vi "C884Config.vi"(0 "All axes? Refnum":refnum<vi>, 1 "Stage selection":T2={"Force?"=FALSE, "Dialog?"=TRUE, "Stages"=[]}, 2 "Position Refnum":refnum<vi>, 3 "Identification Refnum":refnum<vi>, 4 "Referencing successful Refnum":refnum<vi>, 5 "Host Addresss Refnum":refnum<vi>, 6 "Message Out Refnum":refnum<vi>, 7 "+/- mvt range Refnum":refnum<vi>, 8 "Axes to Move Refnum":refnum<vi>, 9 "Connected Axes Refnum":refnum<vi>, 10 "Referencing":T1={"Check FRF?"=TRUE, "Referencing mode"=[enum."FRF (-> FNL)", enum."FRF (-> FNL)", enum."FRF (-> FNL)", enum."FRF (-> FNL)", enum."FRF (-> FNL)", enum."FRF (-> FNL)"]}, 11 "Error OUT Refnum":refnum<vi>, 12 "En cours LED Refnum":refnum<vi>, 13 "LED Initialis. OK? Refnum":refnum<vi>) -> ()   [LabVIEW 2013]
panel:
  out "+/- movement\nrange":dbl[](array[numeric]) format="%.6f"
  out "error out":errorcluster
  out "Identification":string
  out "Referencing\nsuccessful?":bool[](array[boolean])
  out "Conn. \nAxes":string[](array[string])
  out "Position":dbl[](array[numeric]) format="%.6f"
  out "TCP/IP settings.Host address/name":string
  # "If yes:"
  # "If not:"
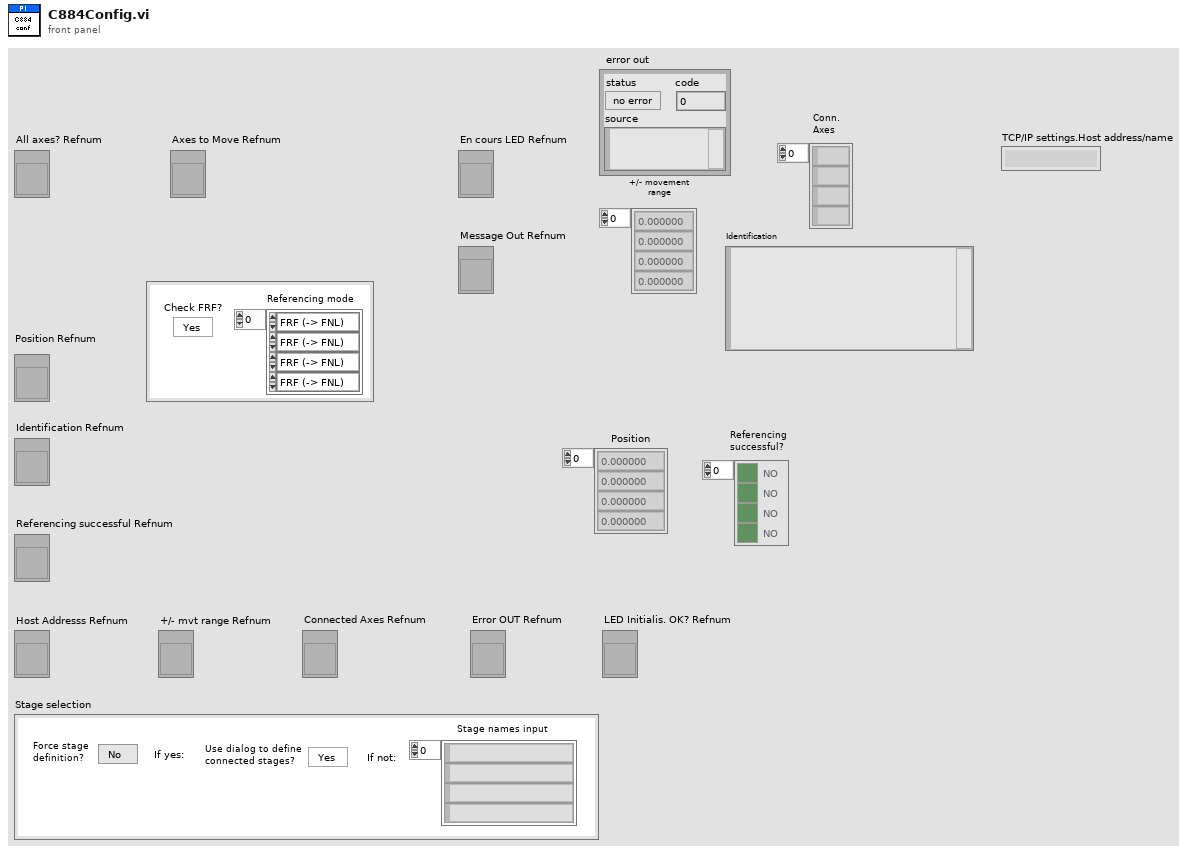
[diagram p1: front panel]
types:
  T1 = cluster{"Check FRF?":bool, "Referencing mode":enum16{"FRF (-> FNL)", "FRF", "FNL", "FPL", "RON OFF"}[]}
  T2 = cluster{"Force?":bool, "Dialog?":bool, "Stages":string[]}
  T3 = cluster{"RS232 settings":cluster{"Portnumber":i32, "Baudrate":u16}, "TCP/IP settings":cluster{"Host address/name":string, "Port":i32, "Board":i32, "TCP/IP Search?":bool}, "USB settings":cluster{"S/N":string, "USB Search?":bool}}
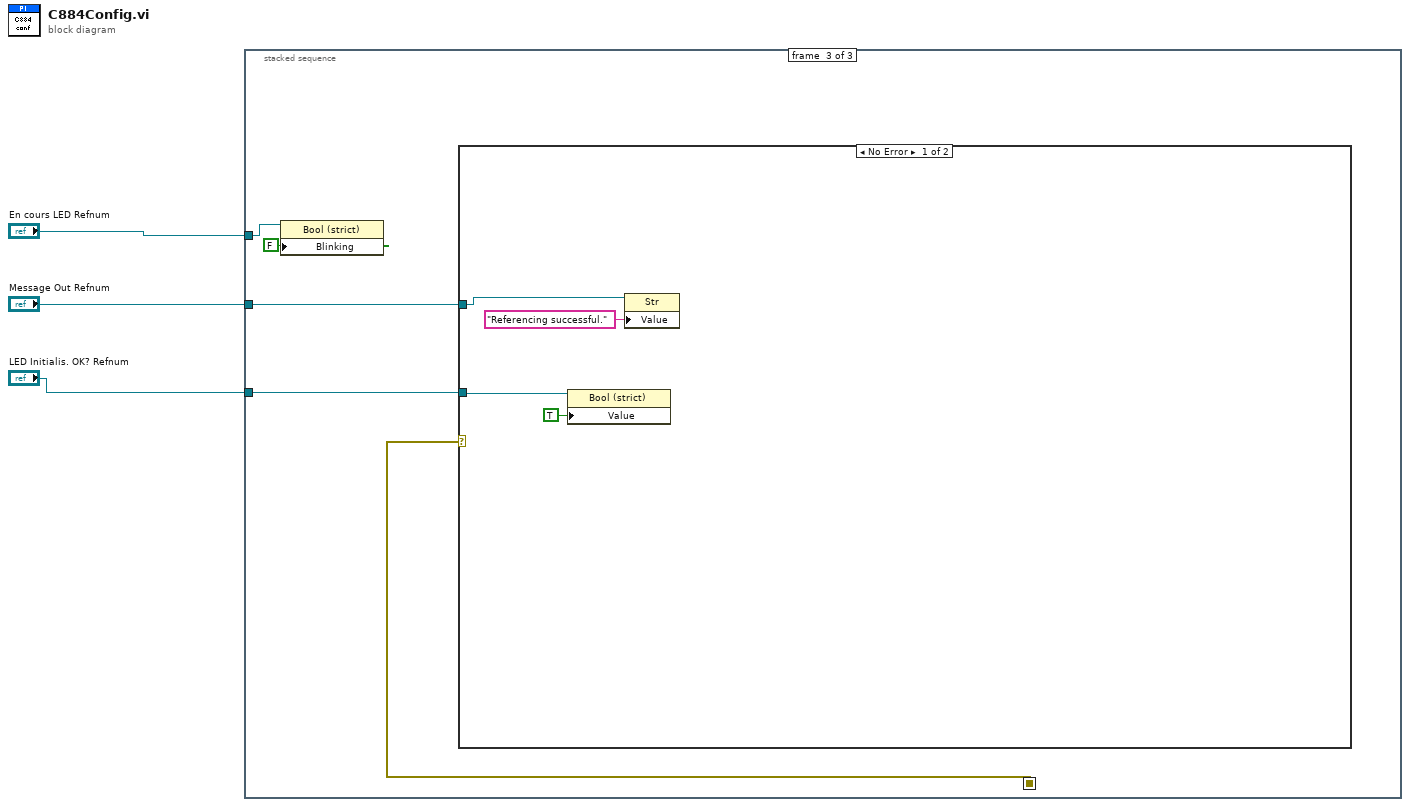
[diagram p0: block diagram]
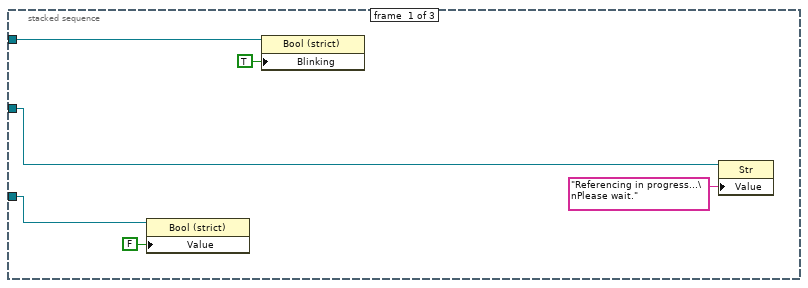
[diagram p2: hidden frame]
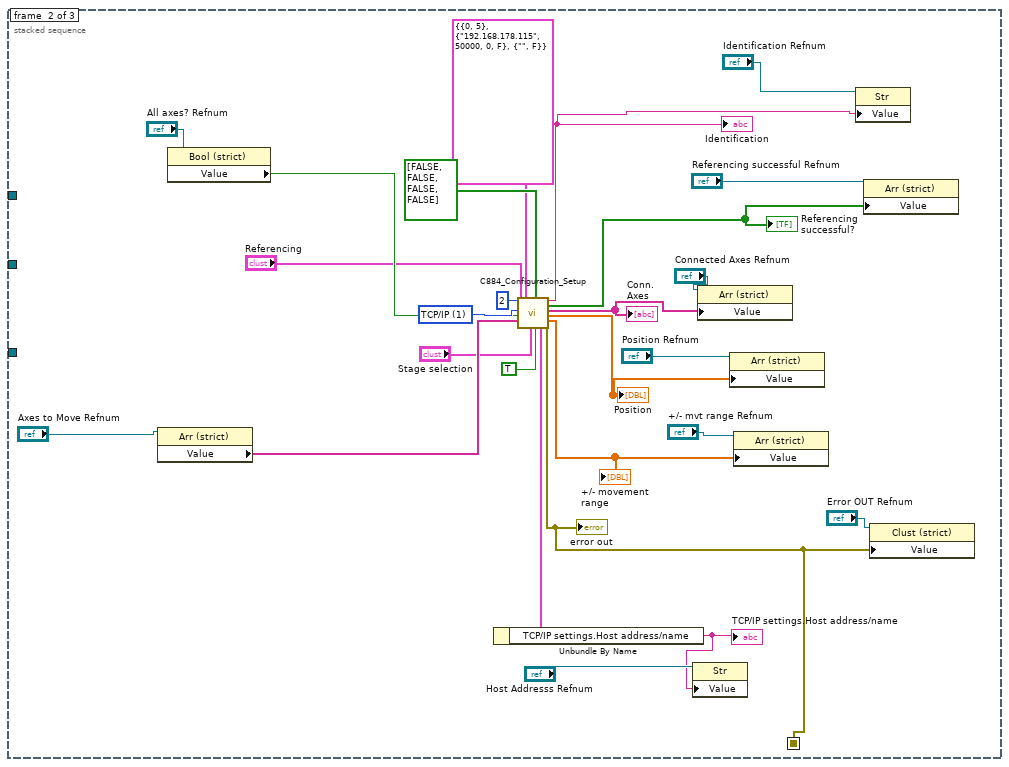
[diagram p3: hidden frame]
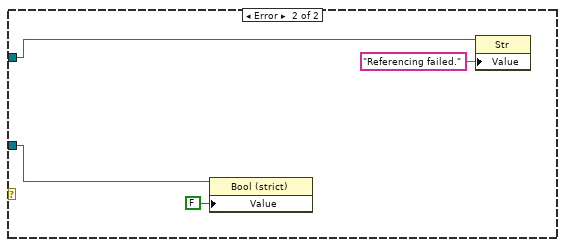
[diagram p4: hidden frame]
diagram:
  n1 = stacked-sequence {
    seq-local: [_ w14 _] -> [_ _ w38]
    tunnel: "En cours LED Refnum" -> [w8 _ w39]
    tunnel: "Message Out Refnum" -> [w7 _ w37]
    tunnel: "LED Initialis. OK? Refnum" -> [w5 _ w36]
    frame #0 {
      n2 = property class="Bool (strict)"(reference=w5, "Value"=FALSE) -> ()  [unwired: 1 in, 2 out]
      n3 = property class="Bool (strict)"(reference=w8, "Blinking"=TRUE) -> ()  [unwired: 1 in, 2 out]
      n4 = property class="Str"(reference=w7, "Value"="Referencing in progress...\nPlease wait.") -> ()  [unwired: 1 in, 2 out]
    }
    frame #1 {
      w32 = u16 1 items=["RS232", "TCP/IP", "USB"] ("Interface")
      n5 = property class="Arr (strict)"(reference="Axes to Move Refnum") -> ("Value"=w28:string[])  [unwired: 1 in, 2 out]
      n6 = property class="Bool (strict)"(reference="All axes? Refnum") -> ("Value"=w29:bool)  [unwired: 1 in, 2 out]
      n7 = call "C884_Configuration_Setup.vi"("System no."=2, "Referencing"="Referencing", "Interface"=w32, "All axes?"=w29, "Axes to move"=w28, "Interface settings"=T3 {"RS232 settings"={"Portnumber"=0, "Baudrate"=5}, "TCP/IP settings"={"Host address/name"="192.168.178.115", "Port"=50000, "Board"=0, "TCP/IP Search?"=FALSE}, "USB settings"={"S/N"="", "USB Search?"=FALSE}}, "Stage selection"="Stage selection", "Move to middle?"=bool[] [FALSE, FALSE, FALSE, FALSE], "Switch servo on?"=TRUE) -> ("Interface settings out"=w33:T3, "Identification"=w15:string, "Referencing\nsuccessful?"=w17:bool[], "Conn. \nAxes"=w19:string[], "Position"=w21:dbl[], "+/- movement\nrange"=w23:dbl[], "error out"=w14:errorcluster)  [unwired: 4 in]
      "Position" <- w21
      "Conn. \nAxes" <- w19
      "Referencing\nsuccessful?" <- w17
      "Identification" <- w15
      "error out" <- w14
      "+/- movement\nrange" <- w23
      n8 = Unbundle By Name(w33) -> ("TCP/IP settings.Host address/name"=w26:string)
      "TCP/IP settings.Host address/name" <- w26
      n9 = property class="Str"(reference="Host Addresss Refnum", "Value"=w26) -> ()  [unwired: 1 in, 2 out]
      n10 = property class="Arr (strict)"(reference="Connected Axes Refnum", "Value"=w19) -> ()  [unwired: 1 in, 2 out]
      n11 = property class="Arr (strict)"(reference="Position Refnum", "Value"=w21) -> ()  [unwired: 1 in, 2 out]
      n12 = property class="Arr (strict)"(reference="+/- mvt range Refnum", "Value"=w23) -> ()  [unwired: 1 in, 2 out]
      n13 = property class="Str"(reference="Identification Refnum", "Value"=w15) -> ()  [unwired: 1 in, 2 out]
      n14 = property class="Arr (strict)"(reference="Referencing successful Refnum", "Value"=w17) -> ()  [unwired: 1 in, 2 out]
      n15 = property class="Clust (strict)"(reference="Error OUT Refnum", "Value"=w14) -> ()  [unwired: 1 in, 2 out]
    }
    frame #2 {
      n16 = property class="Bool (strict)"(reference=w39, "Blinking"=FALSE) -> ()  [unwired: 1 in, 2 out]
      n17 = case shown="No Error" w38 {
        tunnel: w37 -> [w44 w47]
        tunnel: w36 -> [w41 w45]
        frame No Error {
          n18 = property class="Bool (strict)"(reference=w41, "Value"=TRUE) -> ()  [unwired: 1 in, 2 out]
          n19 = property class="Str"(reference=w44, "Value"="Referencing successful.") -> ()  [unwired: 1 in, 2 out]
        }
        frame Error {
          n20 = property class="Bool (strict)"(reference=w45, "Value"=FALSE) -> ()  [unwired: 1 in, 2 out]
          n21 = property class="Str"(reference=w47, "Value"="Referencing failed.") -> ()  [unwired: 1 in, 2 out]
        }
      }
    }
  }
